vi "Loop_Send to Dashboard.vi"() -> ()   [LabVIEW 2017, in "DashBoardCom.lvlib"]
uses:
  DashBoardCom.lvlib
  Shared Code/TypeDefs/Cluster_RIO to DashBoard Controls.ctl
  <vilib>/Rock Robotics/WPI/Solenoid/WPI_SolenoidValue.ctl
  _SHARE ALL/Global Share All/Global_STOP.vi
  MechamumDrive/Global_CMD to SM Data.vi
  Shooter/Global_SM_Data Out.vi
  Sonar/Global_HW_Data Out.vi
  Globals/Global_Main CPU Percent.vi
  Gear/Global_GearPistonsCTRL.vi
  MechamumDrive/MechamunDrive.lvlib
  Shooter/Shooter.lvlib
  Sonar/Sonar.lvlib
  Gear/Gear.lvlib
panel:
  out "Data to DB":T1
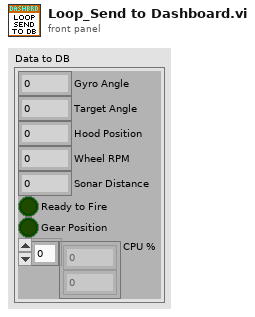
[diagram p1: front panel]
types:
  T1 = typedef "Cluster_RIO to DashBoard Controls.ctl" = cluster{"Gyro Angle":dbl, "Target Angle":dbl, "Hood Position":dbl, "Wheel RPM":dbl, "Sonar Distance":dbl, "Ready to Fire":bool, "Gear Position":bool, "CPU %":dbl[]}
  T2 = typedef "WPI_SolenoidValue.ctl" = enum16{"Off", "On", "Forward", "Reverse"}
  T3 = cluster{"Total (%)":dbl, "Time Critical (%)":dbl, "Timed Structures (%)":dbl, "High (%)":dbl, "Above Normal (%)":dbl, "Normal (%)":dbl, "Background (%)":dbl, "Idle (%)":dbl, "ISR (%)":dbl}[]
  T4 = typedef "Shooter.lvlib/Cluster_SM to HW Wheel Data.ctl" = cluster{"Use Encoder":bool, "VBus":dbl, "RPM":dbl}
  T5 = typedef "Shooter.lvlib/Cluster_SM to HW Hood Data.ctl" = cluster{"Use Encoder":bool, "VBus":dbl, "Position":dbl}
  T6 = typedef "MechamunDrive.lvlib/Cluster_CMD to SM Data.ctl" = cluster{"CMDMODE":T7, "X":dbl, "Y":dbl, "Rotation":dbl, "Auto Angle":dbl, "Speed Divider":dbl, "Use Gyro":bool, "Target Distance":dbl}
  T7 = typedef "MechamunDrive.lvlib/Enum_SM Cmd Select.ctl" = enum16{"No Command", "Halt", "Manual Keep Rotation", "Manual", "Track Front", "Track Rotation", "Track Lateral", "Track Vision Lat", "Track Vision Rot", "Strafe Right", "Strafe Left"}
  T8 = cluster{"Total (%)":dbl, "Time Critical (%)":dbl, "Timed Structures (%)":dbl, "High (%)":dbl, "Above Normal (%)":dbl, "Normal (%)":dbl, "Background (%)":dbl, "Idle (%)":dbl, "ISR (%)":dbl}
  T9 = cluster{"Yaw":dbl, "Roll":dbl, "Pitch":dbl, "Heading":dbl, "Fused Heading":dbl}
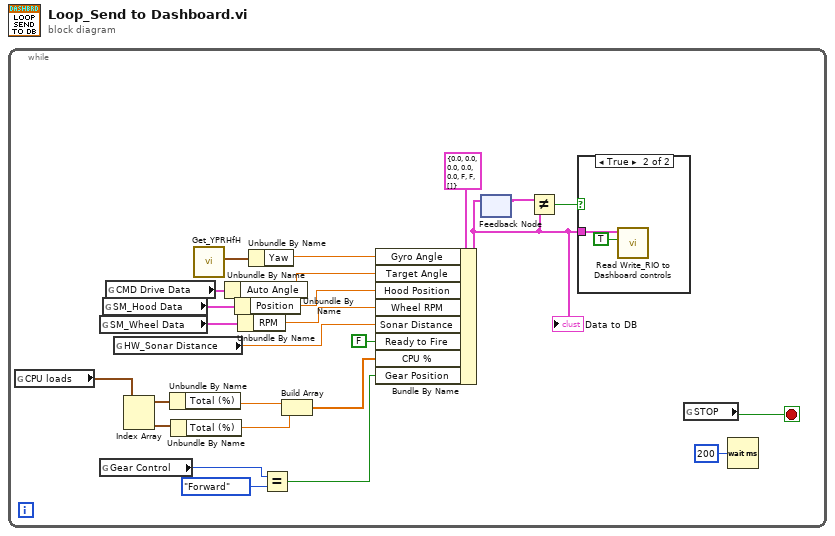
[diagram p0: block diagram]
diagram:
  n1 = while {
    stop <- w24 stop-if-true
    n2 = global read "Global_Main CPU Percent.vi" "CPU loads"() -> (w9:T3)
    n3 = global read "Global_SM_Data Out.vi" "SM_Wheel Data"() -> (w13:T4)
    n4 = global read "Global_GearPistonsCTRL.vi" "Gear Control"() -> (w3:T2)
    n5 = global read "Global_SM_Data Out.vi" "SM_Hood Data"() -> (w15:T5)
    n6 = global read "Global_CMD to SM Data.vi" "CMD Drive Data"() -> (w17:T6)
    n7 = global read "Global_HW_Data Out.vi" "HW_Sonar Distance"() -> (w11:dbl)
    n8 = Index Array(array=w9) -> (element #1=w8:T8, element #2=w7:T8)  [unwired: 2 in]
    n9 = Unbundle By Name(w8) -> ("Total (%)"=w6:dbl)
    n10 = Unbundle By Name(w7) -> ("Total (%)"=w5:dbl)
    n11 = call <vilib>:"Get_YPRHfH.vi"() -> ("YRPHfH"=w19:T9)  [unwired: 11 in]
    n12 = Unbundle By Name(w17) -> ("Auto Angle"=w16:dbl)
    n13 = Unbundle By Name(w15) -> ("Position"=w14:dbl)
    n14 = Unbundle By Name(w13) -> ("RPM"=w12:dbl)
    n15 = Unbundle By Name(w19) -> ("Yaw"=w18:dbl)
    n16 = Equal?(x=w3, y=WPI_SolenoidValue."Forward") -> (x = y?=w1:bool)
    n17 = Build Array(w6, w5) -> (w4:dbl[])
    n18 = Bundle By Name(cluster=T1 {"Gyro Angle"=0.0, "Target Angle"=0.0, "Hood Position"=0.0, "Wheel RPM"=0.0, "Sonar Distance"=0.0, "Ready to Fire"=FALSE, "Gear Position"=FALSE, "CPU %"=[]} ("Data In"), "Gyro Angle"=w18, "Target Angle"=w16, "Hood Position"=w14, "Wheel RPM"=w12, "Sonar Distance"=w11, "Ready to Fire"=FALSE, "CPU %"=w4, "Gear Position"=w1) -> (w20:T1)
    "Data to DB" <- w20
    n19 = feedback-in #1(w20) -> ()
    n20 = feedback #1() -> (w23:T1)  [unwired: 1 in]
    n21 = Not Equal?(x=w23, y=w20) -> (x != y?=w22:bool)
    n22 = case shown="True" w22 {
      tunnel: w20 -> [_ w26]
      frame False {
      }
      frame True {
        n23 = call "Read Write_RIO to Dashboard controls.vi"("Read(F) Write(T)"=TRUE, "Data In"=w26) -> ()  [unwired: 9 in, 1 out]
      }
    }
    n24 = global read "Global_STOP.vi" "STOP"() -> (w24:bool)
    n25 = Wait (ms)(milliseconds to wait=u32 200) -> ()  [unwired: 1 out]
  }
